vi "TestMFCLegacy.vi"() -> ()   [LabVIEW 2018]
panel:
  out "Legacy Status":u8(ring) items=["Rev. 21 Board", "Rev. 22 Board", "Rev. 23 Board"]
  out "error out":errorcluster
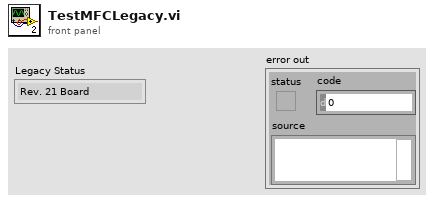
[diagram p1: front panel]
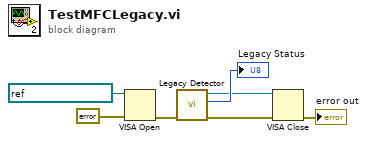
[diagram p0: block diagram]
diagram:
  n1 = VISA Open(error in (no error)=errorcluster {"status"=FALSE, "code"=0, "source"=""}, VISA resource name=refnum<visa-resource-name> "OpticalShutter") -> (error out=w6:errorcluster)  [unwired: 3 in, 1 out]
  n2 = call "Legacy Detector.vi"("error in"=w6) -> ("error out"=w3:errorcluster, "Legacy Status"=→"Legacy Status":u8, "VISA Session Out"=w1:refnum<visa-resource-name>)  [unwired: 8 in]
  n3 = VISA Close(VISA resource name=w1, error in (no error)=w3) -> (error out=→"error out":errorcluster)
